vi "get paired node.vi"(8 "error in":errorcluster, 11 "editor in":refnum<data-value>) -> (0 "error out":errorcluster, 2 "paired node":refnum<data-value>, 3 "editor out":refnum<data-value>)   [LabVIEW 2013, in "TEC editor node.lvclass"]
uses:
  TEC editor node.lvclass
  <vilib>/NI/Tag Bus Module Framework/root configuration/TBM configuration.lvclass/TBM configuration.ctl
  <vilib>/NI/Tag Bus Module Framework/root configuration/Read instance name.vi
  read pair information.vi
  <vilib>/NI/Tag Bus Module Framework/root configuration/create GUID.vi
  <vilib>/NI/Tag Bus Module Framework/root configuration/TBM configuration.lvclass
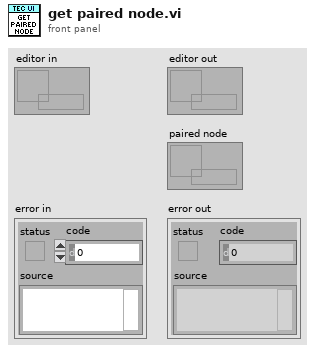
[diagram p1: front panel]
types:
  T1 = typedef "TEC editor node.lvclass/pair information.ctl" = cluster{"paired guid":string, "pair type":T2}
  T2 = typedef "TEC editor node.lvclass/pair type.ctl" = enum16{"master", "slave"}
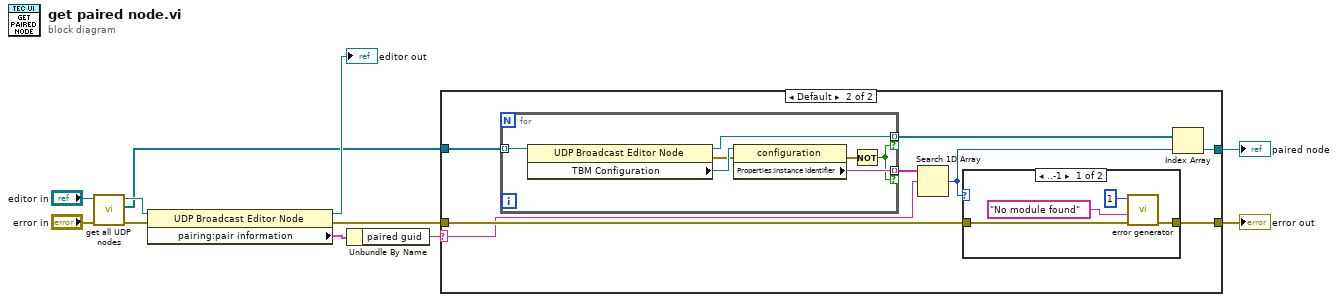
[diagram p0: block diagram]
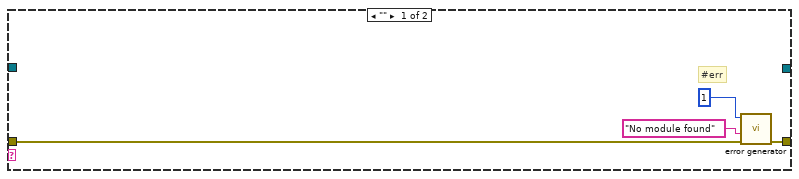
[diagram p2: hidden frame]
diagram:
  n1 = call "get all UDP nodes.vi"("error in"="error in", "editor in"="editor in") -> ("error out"=w5:errorcluster, "All UDP refs"=w1:refnum<data-value>[], "editor out"=w4:refnum<data-value>)  [unwired: 7 in]
  n2 = property class="UDP Broadcast Editor Node"(reference=w4, error in=w5) -> (reference out=→"editor out":refnum<data-value>, error out=w11:errorcluster, "pairing:pair information"=w9:T1)
  n3 = Unbundle By Name(w9) -> ("paired guid"=w8:string)
  n4 = case shown="Default" w8 {
    selector: w8 -> [_ w21]
    tunnel: w11 -> [w15 w23]
    tunnel: [w14 w17] -> w10
    tunnel: [_ w19] -> w7
    tunnel: w1 -> [_ w16]
    frame "" {
      # "#err"
      n5 = call <vilib>:"error generator.vi"("error in"=w15, "source"="No module found", "error code (0)"=1) -> ("error out"=w14:errorcluster)  [unwired: 8 in]
    }
    frame Default {
      n6 = for {
        tunnel: w16 -> [w35] mode=indexing
        tunnel: [w32] -> w22 mode=indexing if=w29
        tunnel: [w30] -> w20 mode=indexing if=w29
        n7 = property class="UDP Broadcast Editor Node"(reference=w35) -> (reference out=w30:refnum<data-value>, error out=w33:errorcluster, "TBM Configuration"=w34:refnum<class "TBM configuration.lvclass">)  [unwired: 1 in]
        n8 = property class="configuration"(reference=w34, error in=w33) -> (error out=w31:errorcluster, "Properties:instance identifier"=w32:string)  [unwired: 1 out]
        n9 = Not(x=w31) -> (.not. x?=w29:bool)
      }
      n10 = Search 1D Array(1D array=w22, element=w21) -> (index of element=w18:i32)  [unwired: 1 in]
      n11 = case shown="..-1" w18 {
        tunnel: w23 -> [w25 w28]
        tunnel: [w24 w28] -> w17
        frame ..-1 {
          n12 = call <vilib>:"error generator.vi"("error in"=w25, "source"="No module found", "error code (0)"=1) -> ("error out"=w24:errorcluster)  [unwired: 8 in]
        }
        frame 0.. {
        }
      }
      n13 = Index Array(array=w20, index=w18) -> (element=w19:refnum<data-value>)
    }
  }
  "error out" <- w10
  "paired node" <- w7
